vi "Get Log File Reference.vi"(8 "error in":errorcluster, 10 "Overwrite File If Exists?":bool, 11 "Log File Path":path) -> (0 "error out":errorcluster, 3 "Log File Refnum out":refnum<k34>)   [LabVIEW 2020, in "Telemetry Engine.lvlib"]
doc: "This subVI creates the telemetry.tdms log file used for logging the benchmark data."
uses:
  Telemetry Engine.lvlib
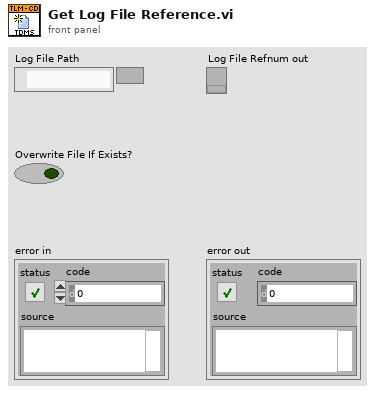
[diagram p1: front panel]
types:
  T1 = enum16{"open", "open or create", "create or replace", "create", "open (read-only)"}
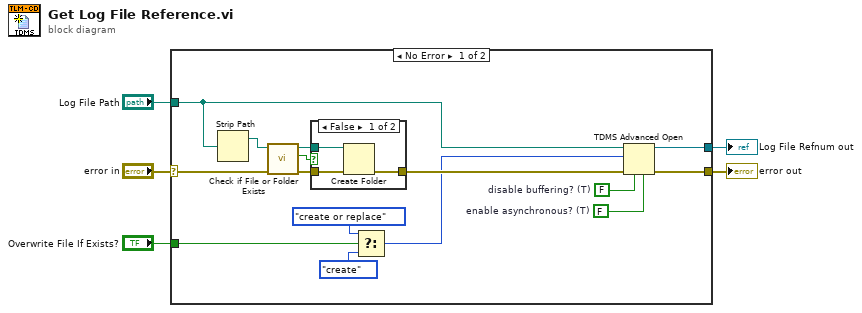
[diagram p0: block diagram]
diagram:
  n1 = case shown="No Error" "error in" {
    selector: "error in" -> [w8 w25]
    tunnel: [w20 w25] -> w5
    tunnel: "Log File Path" -> [w18 _]
    tunnel: "Overwrite File If Exists?" -> [w6 _]
    tunnel: [w7 _] -> w1
    frame No Error {
      w10 = FALSE  # enable asynchronous? (T)
      w9 = FALSE  # disable buffering? (T)
      n2 = Strip Path(path=w18) -> (stripped path=w17:path)  [unwired: 1 out]
      n3 = call <vilib>:"Check if File or Folder Exists.vi"("error in (no error)"=w8, "path"=w17) -> ("error out"=w15:errorcluster, "file or folder exists?"=w14:bool, "dup path"=w19:path)  [unwired: 7 in]
      n4 = case shown="False" w14 {
        tunnel: w15 -> [w23 w24]
        tunnel: [w22 w24] -> w16
        tunnel: w19 -> [w21 _]
        frame False {
          n5 = Create Folder(path (use dialog)=w21, error in=w23) -> (error out=w22:errorcluster)  [unwired: 1 in, 2 out]
        }
        frame True {
        }
      }
      n6 = Select(t=T1."create or replace" ("operation (0:open)"), s=w6, f=T1."create" ("operation (0:open)")) -> (s? t:f=w13:T1)
      n7 = TDMS Advanced Open(4:w10, 6:w9, 8:w16, 10:w13, 11:w18) -> (0:w20:errorcluster, 3:w7:refnum<k34>)  [unwired: 1 out]
    }
    frame Error {
    }
  }
  "Log File Refnum out" <- w1
  "error out" <- w5
